vi "Robot Global Data.vi"() -> ()   [LabVIEW 2015]
doc: "This global VI can contain as many global variables as you need. Place a control on the panel, give it a good name. To read or write to it from a VI, drag the icon to the diagram of that VI. You can also drag from the project. Click on the node to change which global you access. You shouldn't have multiple locations writing to a global or it will cause a race-condition."
uses:
  <vilib>/Rock Robotics/WPI/Camera/WPI_CameraImageSize.ctl
  <vilib>/Rock Robotics/WPI/DriverStation/WPI_DriverStationRobotMode2.ctl
panel:
  out "Gyro Error":dbl
  out "Auto Position":dbl
  out "Gyro Drift":dbl
  out "Right Encoder":dbl
  out "Left Encoder":dbl
  in  "PID Auto Fire":bool
  out "BottomHall":bool
  out "TopHall":bool
  in  "BottomPot":dbl
  in  "TopPot":dbl
  out "Got Vision Packet?":bool
  out "AimArray":dbl[][](array[numeric])
  out "Request Vision Packet":bool
  in  "Numeric":dbl
  in  "Don't touch!":T1
  in  "Aiming Data":T2
  in  "Current Gear":bool
  in  "Automatic Shifting":bool
  out "Gyro Angle":dbl
  out "Vision Data":T3
  out "Gyro Correction":dbl
  out "Gyro Setpoint":dbl
  in  "Robot Mode":T4
  in  "image size":T5=enum."320x240"
  in  "Enable Vision":bool
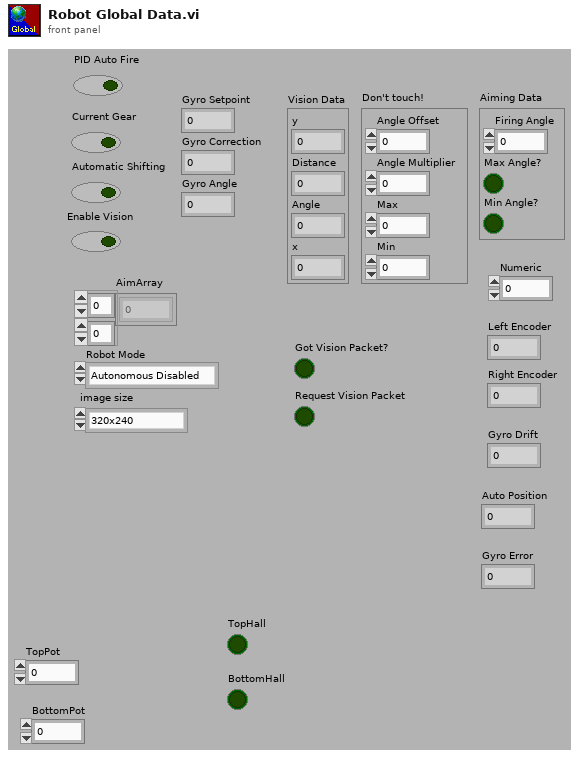
[diagram p1: front panel]
types:
  T1 = cluster{"Angle Offset":dbl, "Angle Multiplier":dbl, "Max":dbl, "Min":dbl}
  T2 = cluster{"Firing Angle":dbl, "Max Angle?":bool, "Min Angle?":bool}
  T3 = cluster{"y":dbl, "Distance":dbl, "Angle":dbl, "x":dbl}
  T4 = typedef "WPI_DriverStationRobotMode2.ctl" = enum16{"Autonomous Disabled", "Autonomous Enabled", "Teleop Disabled", "Teleop Enabled", "Disconnected", "Finish", "Test Disabled", "Test Enabled", "Emergency Stopped"}
  T5 = typedef "WPI_CameraImageSize.ctl" = enum16{"640x480", "320x240", "160x120", "Custom"}
diagram:
